vi "setBarPalette.vi"(8 "Error In":errorcluster, 10 "palette":refnum<class "QPalette.lvclass">, 11 "LQwtPlotBarChart In":refnum<class "LQwtPlotBarChart.lvclass">) -> (0 "Error Out":errorcluster, 3 "LQwtPlotBarChart Out":refnum<class "LQwtPlotBarChart.lvclass">)   [LabVIEW 2014, in "LQwtPlotBarChart.lvclass"]
doc: "LabVIEW-specific documentation is not yet available."
uses:
  LQwtPlotBarChart.lvclass
  Qt GUI/QPalette/QPalette.lvclass
  LQ Core/LQIdentity/LQIdentity.lvclass/LQIdentity.ctl
  LQ Core/LQSerialData/LQSerialData.lvclass/LQSerialData.ctl
  LQ Core/LQ Core.lvlib
  LQ Core/LQIdentity/LQIdentity.lvclass
  LQ Core/LQSerialData/LQSerialData.lvclass
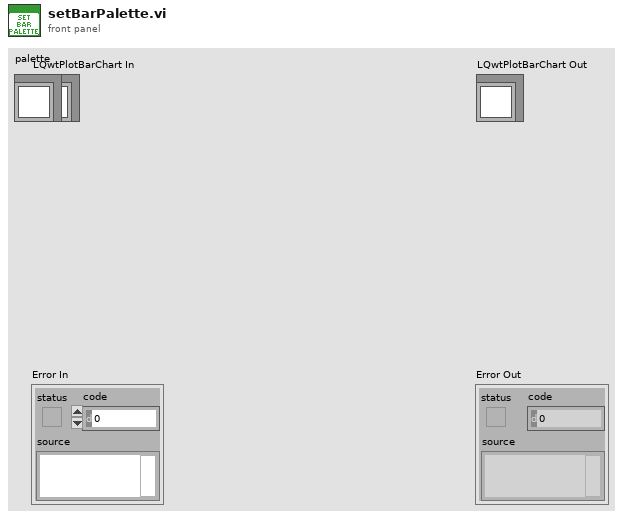
[diagram p1: front panel]
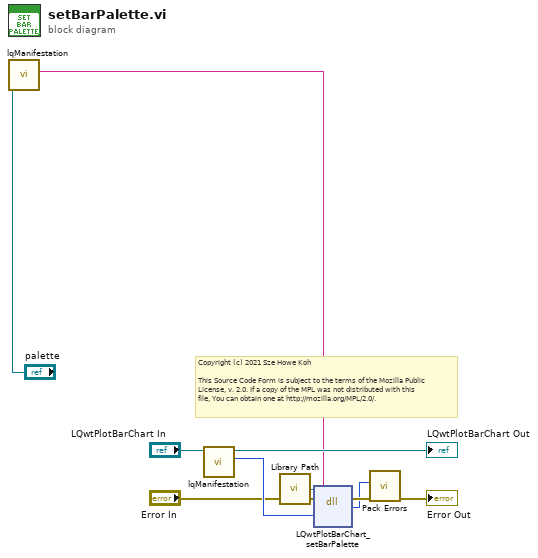
[diagram p0: block diagram]
diagram:
  # "Copyright (c) 2021 Sze Howe Koh\n\nThis Source Code Form is subject to the terms of the Mozilla Public\nLicense, v. 2.0. If a copy of the MPL was not distributed with this\nfile, You can obtain one at http://mozilla.org/MPL/2.0/."
  n1 = call "lqManifestation.vi"("LQSerialData in"="palette") -> ("Manifestation"=w1:string)  [unwired: 9 in, 1 out]
  n2 = call "lqManifestation.vi"("LQIdentity in"="LQwtPlotBarChart In") -> ("Manifestation"=w7:u64, "LQIdentity out"=→"LQwtPlotBarChart Out":refnum<class "LQwtPlotBarChart.lvclass">)  [unwired: 9 in]
  n3 = call "Library Path.vi"() -> ("Library Path"=w8:path)
  n4 = dll-call lib="?" fn="LQwtPlotBarChart_setBarPalette"(path in=w8, error in="Error In", "_instance"=w7, "palette"=w1) -> (error out=w5:errorcluster, w3:i32)  [unwired: 3 in, 1 out]
  n5 = call "Pack Errors.vi"("Error In"=w5, "Error Code"=w3) -> ("Error Out"=→"Error Out":errorcluster)  [unwired: 9 in]
